vi "TcA01-009_ObjectCreationWithNoRegistration.vi"(1 "Input buffer":T3="1", 3 "Invocation info":T2, 5 "error in (no error)":errorcluster, 6 "Add log to result?":bool) -> (16 "Test Data":T1 {"Numeric Measurement" format="%.2f"}, 19 "error out":errorcluster)   [LabVIEW 2020]
doc: "Test case template."
uses:
  Shared/Support_InputBuffer.ctl
  Shared/Support_InvocationInfo.ctl
  Shared/Support_TestData.ctl
  TestClasses/G#SubClass1_class/G#SubClass1.lvclass
  <vilib>/addons/_AddQ/G#Object/G#Object.lvclass
panel:
  in  "Test name":string="TcA01-009 Object creation with no registration"
  out "Test result":bool
  out "Result":string
  # "Verify that objects with no registration works."
  # "Sub test case"
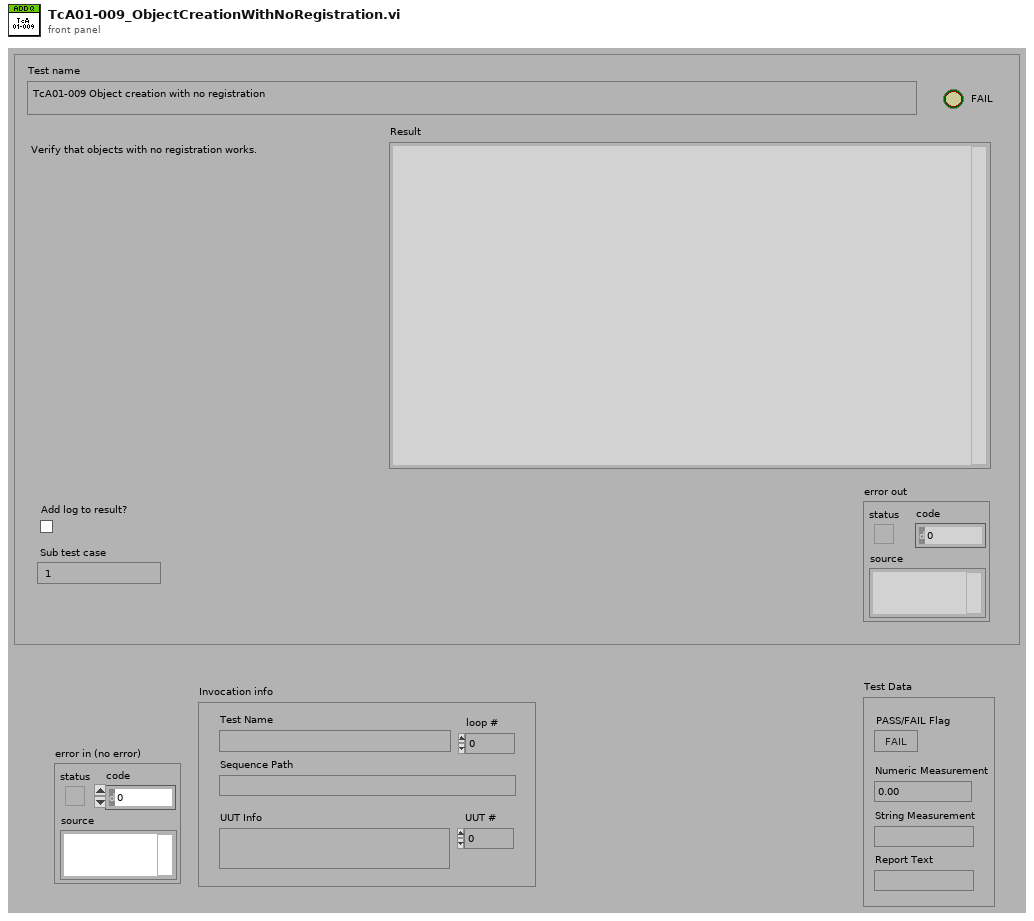
[diagram p1: front panel]
types:
  T1 = typedef "Support_TestData.ctl" = cluster{"PASS/FAIL Flag":bool, "Numeric Measurement":dbl, "String Measurement":string, "Report Text":string}
  T2 = typedef "Support_InvocationInfo.ctl" = cluster{"UUT #":i32, "loop #":i32, "UUT Info":string, "Test Name":string, "Sequence Path":path}
  T3 = typedef "Support_InputBuffer.ctl" = string
  T4 = typedef "Support_ResultType.ctl" = cluster{"Pass":bool, "Comment":string, "MeasurementValue":dbl}
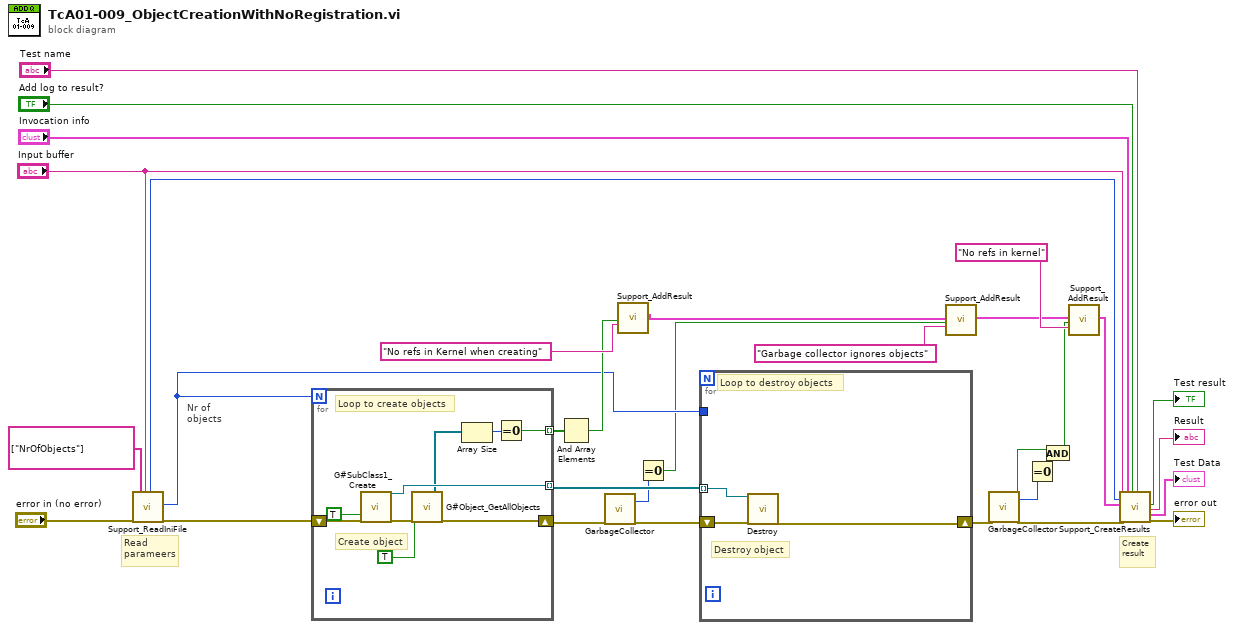
[diagram p0: block diagram]
diagram:
  # "Read\nparameers"
  # "Create\nresult"
  # "Nr of\nobjects"
  n1 = call "Support_ReadIniFile.vi"("error in (no error)"="error in (no error)", "Parameter names"=string[] ["NrOfObjects"], "Sub test case"="Input buffer") -> ("Timer start"=w18:u32, "Parameter1 as I32"=w8:i32, "error out"=w1:errorcluster)  [unwired: 9 in, 5 out]
  n2 = for {
    N: w8 -> [_]
    shift-right: [w36] -> w5
    shift-left: w1 -> [w41]
    tunnel: [w39] -> w22 mode=indexing
    tunnel: [w34] -> w25 mode=indexing
    # "Create object"
    # "Loop to create objects"
    n3 = call "G#SubClass1_Create.vi"("no registration"=TRUE, "error in (no error)"=w41) -> ("reference out"=w39:refnum<class "G#SubClass1.lvclass">, "error out"=w40:errorcluster)  [unwired: 15 in, 1 out]
    n4 = call <vilib>:"G#Object_GetAllObjects.vi"("only refs (F)"=TRUE ("only refs"), "error in (no error)"=w40) -> ("all refs"=w38:refnum<class "G#Object.lvclass">[], "error out"=w36:errorcluster)  [unwired: 14 in, 2 out]
    n5 = Array Size(array=w38) -> (size(s)=w35:i32)
    n6 = Equal To 0?(x=w35) -> (x = 0?=w34:bool)
  }
  n7 = And Array Elements(Boolean array=w25) -> (logical AND=w23:bool)
  n8 = call <vilib>:"GarbageCollector.vi"("error in (no error)"=w5) -> ("# of objects killed"=w3:i32, "error out"=w4:errorcluster)  [unwired: 16 in, 1 out]
  n9 = call "Support_AddResult.vi"("Pass"=w23, "Comment"="No refs in Kernel when creating") -> ("Results out"=w17:T4[])  [unwired: 17 in]
  n10 = Equal To 0?(x=w3) -> (x = 0?=w2:bool)
  n11 = for {
    shift-right: [w42] -> w16
    shift-left: w4 -> [w44]
    tunnel: w22 -> [w43] mode=indexing
    tunnel: w8 -> [_]
    # "Destroy object"
    # "Loop to destroy objects"
    n12 = call-dynamic "Destroy.vi"("reference in"=w43, "error in (no error)"=w44) -> ("error out"=w42:errorcluster)  [unwired: 16 in, 1 out]
  }
  n13 = call "Support_AddResult.vi"("Results in"=w17, "Pass"=w2, "Comment"="Garbage collector ignores objects") -> ("Results out"=w6:T4[])  [unwired: 16 in]
  n14 = call <vilib>:"GarbageCollector.vi"("error in (no error)"=w16) -> ("OK"=w12:bool, "# of objects killed"=w10:i32, "error out"=w15:errorcluster)  [unwired: 16 in]
  n15 = Equal To 0?(x=w10) -> (x = 0?=w11:bool)
  n16 = And(x=w12, y=w11) -> (x .and. y?=w9:bool)
  n17 = call "Support_AddResult.vi"("Results in"=w6, "Pass"=w9, "Comment"="No refs in kernel") -> ("Results out"=w14:T4[])  [unwired: 16 in]
  n18 = call "Support_CreateResults.vi"("Sub test case"="Input buffer", "Timer start"=w18, "Results"=w14, "error in (no error)"=w15, "Invocation info"="Invocation info", "Add log to result?"="Add log to result?", "Test name"="Test name") -> ("Pass/fail flag"=→"Test result":bool, "Result"=→"Result":string, "Test Data"=→"Test Data":T1, "error out"=→"error out":errorcluster)  [unwired: 9 in]
